vi "Array with random number.vi"() -> ()   [LabVIEW 2011]
panel:
  out "Array":dbl[][][](array[numeric]) format="%#.2g"
  # "Run the VI"
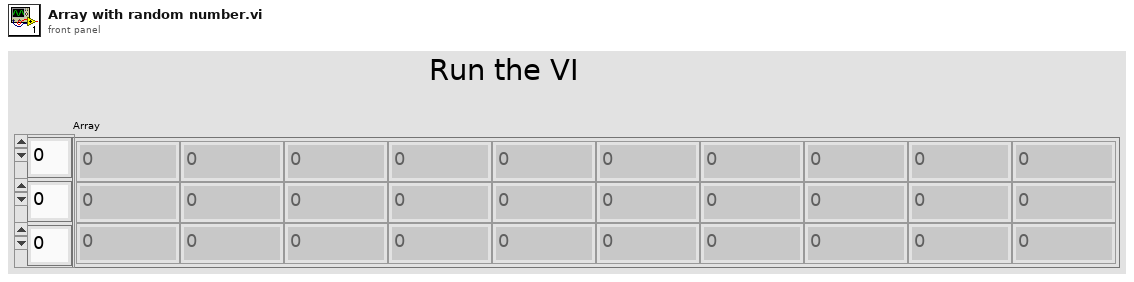
[diagram p1: front panel]
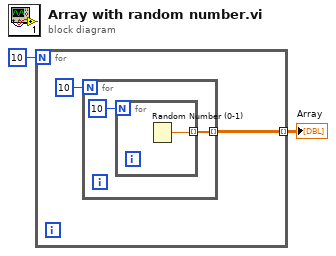
[diagram p0: block diagram]
diagram:
  n1 = for {
    N: 10 -> [_]
    tunnel: [w3] -> w1 mode=indexing
    n2 = for {
      N: 10 -> [_]
      tunnel: [w5] -> w3 mode=indexing
      n3 = for {
        N: 10 -> [_]
        tunnel: [w7] -> w5 mode=indexing
        n4 = Random Number (0-1)() -> (number: 0 to 1=w7:dbl)
      }
    }
  }
  "Array" <- w1
